vi "Set Timeout (ms).vi"(8 "error in (no error)":errorcluster caption="entrée d'erreur (pas d'erreur)", 10 "Timeout (ms)":u64, 11 "Wait_OpenFixture en entrée":refnum<class "Wait_OpenFixture.lvclass">) -> (0 "error out":errorcluster caption="sortie d'erreur", 3 "Wait_OpenFixture en sortie":refnum<class "Wait_OpenFixture.lvclass">)   [LabVIEW 2020, in "Library Test.lvlib" / "Wait_OpenFixture.lvclass"]
uses:
  Wait_OpenFixture.lvclass
  Wait_OpenFixture.lvclass/Wait_OpenFixture.ctl
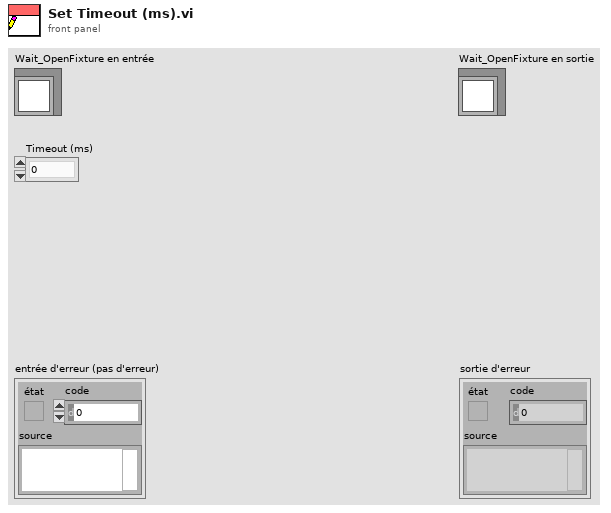
[diagram p1: front panel]
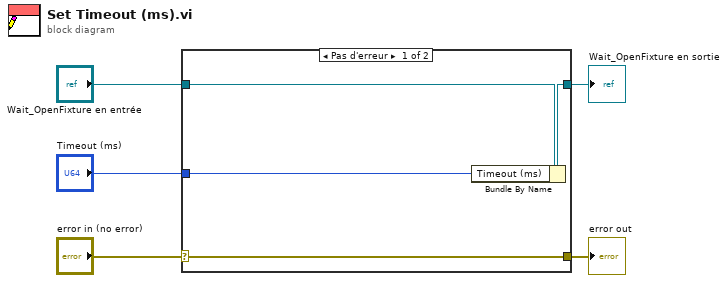
[diagram p0: block diagram]
diagram:
  n1 = case shown="Pas d'erreur" "error in (no error)" {
    selector: "error in (no error)" -> [w9 w10]
    tunnel: [w9 w10] -> w4
    tunnel: [w7 w11] -> w2
    tunnel: "Wait_OpenFixture en entrée" -> [w8 w11]
    tunnel: "Timeout (ms)" -> [w6 _]
    frame No Error {
      n2 = Bundle By Name(cluster=w8, "Timeout (ms)"=w6) -> (w7:refnum<class "Wait_OpenFixture.lvclass">)
    }
    frame Error {
    }
  }
  "error out" <- w4
  "Wait_OpenFixture en sortie" <- w2
